vi "Force circular In Range (DBL).vi"(7 "Max":dbl, 10 "Min":dbl, 11 "Value":dbl) -> (2 "Offset Out":dbl, 3 "Value Out":dbl)   [LabVIEW 2023, in "Thor-SwerveDrive_ACT.lvlib"]
uses:
  Thor-SwerveDrive_ACT.lvlib
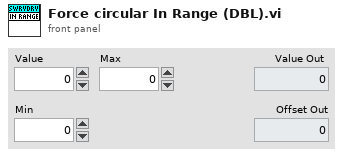
[diagram p1: front panel]
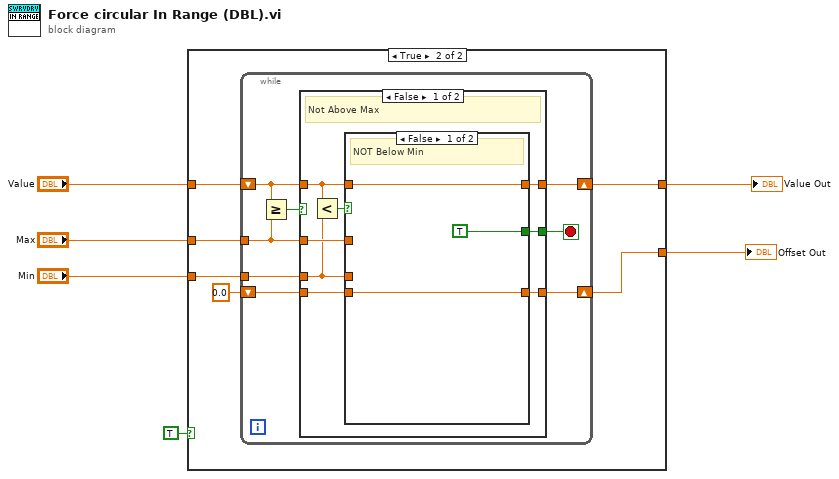
[diagram p0: block diagram]
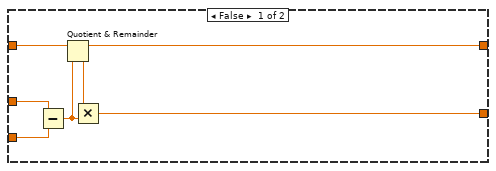
[diagram p2: hidden frame]
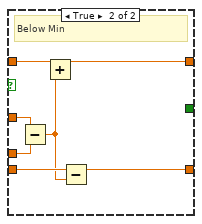
[diagram p3: hidden frame]
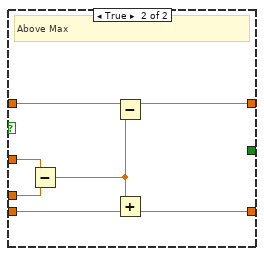
[diagram p4: hidden frame]
diagram:
  n1 = case shown="True" TRUE {
    tunnel: [w7 w19] -> w6
    tunnel: "Value" -> [w11 w18]
    tunnel: "Max" -> [w13 w17]
    tunnel: "Min" -> [w12 w16]
    tunnel: [w8 w15] -> w2
    frame False {
      n2 = Subtract(x=w13, y=w12) -> (x-y=w10:dbl)
      n3 = Quotient & Remainder(x=w11, y=w10) -> (x-y*floor(x/y)=w7:dbl, floor(x/y)=w9:dbl)
      n4 = Multiply(x=w9, y=w10) -> (x*y=w8:dbl)
    }
    frame True {
      n5 = while {
        tunnel: w17 -> [w25]
        shift-right: [w24] -> w19
        shift-left: w18 -> [w26]
        tunnel: w16 -> [w23]
        shift-right: [w20] -> w15
        shift-left: 0.0 -> [w21]
        stop <- w22 stop-if-true
        n6 = Greater Or Equal?(x=w26, y=w25) -> (x >= y?=w27:bool)
        n7 = case shown="False" w27 {
          tunnel: w26 -> [w34 w52]
          tunnel: w25 -> [w33 w49]
          tunnel: [w32 w51] -> w24
          tunnel: w23 -> [w30 w50]
          tunnel: [w31 _] -> w22
          tunnel: w21 -> [w29 w48]
          tunnel: [w28 w47] -> w20
          frame False {
            # "Not Above Max"
            n8 = Less?(x=w34, y=w30) -> (x < y?=w35:bool)
            n9 = case shown="False" w35 {
              tunnel: w34 -> [w38 w45]
              tunnel: w33 -> [_ w42]
              tunnel: [w38 w44] -> w32
              tunnel: [TRUE _] -> w31
              tunnel: w30 -> [_ w43]
              tunnel: w29 -> [w36 w40]
              tunnel: [w36 w41] -> w28
              frame False {
                # "NOT Below Min"
              }
              frame True {
                # "Below Min"
                n10 = Subtract(x=w42, y=w43) -> (x-y=w39:dbl)
                n11 = Add(x=w45, y=w39) -> (x+y=w44:dbl)
                n12 = Subtract(x=w40, y=w39) -> (x-y=w41:dbl)
              }
            }
          }
          frame True {
            # "Above Max"
            n13 = Subtract(x=w49, y=w50) -> (x-y=w46:dbl)
            n14 = Subtract(x=w52, y=w46) -> (x-y=w51:dbl)
            n15 = Add(x=w46, y=w48) -> (x+y=w47:dbl)
          }
        }
      }
    }
  }
  "Value Out" <- w6
  "Offset Out" <- w2
